vi "Write Channels and optional channel names.vi"(10 "Channels and optional channel names":cluster{"Enabled":bool, "Channel name":string}[](array[cluster])=[{"Enabled"=TRUE, "Channel name"=""}, {"Enabled"=FALSE, "Channel name"=""}, {"Enabled"=FALSE, "Channel name"=""}, {"Enabled"=FALSE, "Channel name"=""}], 11 "Switching Time in":refnum<class "Switching Time.lvclass">) -> (3 "Switching Time out":refnum<class "Switching Time.lvclass">)   [LabVIEW 2020, in "Switching Time.lvclass"]
uses:
  Switching Time.lvclass
  Switching Time.lvclass/Switching Time.ctl
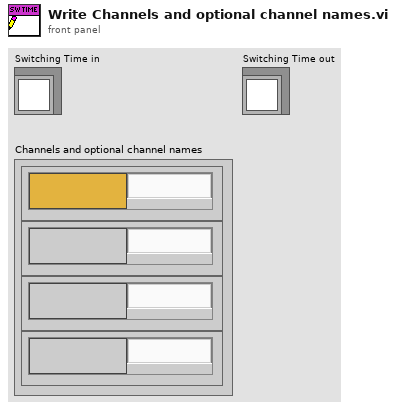
[diagram p1: front panel]
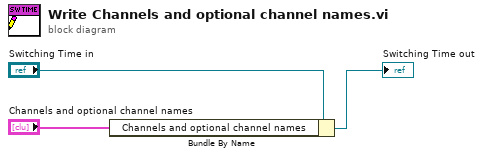
[diagram p0: block diagram]
diagram:
  n1 = Bundle By Name(cluster="Switching Time in", "Channels and optional channel names"="Channels and optional channel names") -> (→"Switching Time out":refnum<class "Switching Time.lvclass">)
